vi "SOFandEOF_del.vi"(8 "error in (no error)":errorcluster, 11 "ISO 14443 B UP in":refnum<class "ISO 14443 B UP.lvclass">) -> (0 "error out":errorcluster, 3 "ISO 14443 B UP out":refnum<class "ISO 14443 B UP.lvclass">)   [LabVIEW 2019, in "ISO 14443 B UP.lvclass"]
uses:
  ISO 14443 B UP.lvclass
  TypeDef/Store.ctl
  ISO 14443 B UP.lvclass/ISO 14443 B UP.ctl
  RFID system.lvclass
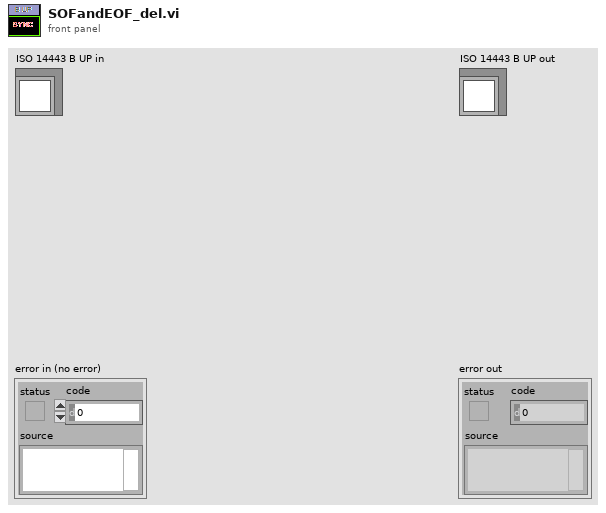
[diagram p1: front panel]
types:
  T1 = typedef "Store.ctl" = enum16{"envelope", "noise", "demSubCar", "CH_frame", "Decode", "demodulate", "in", "out", "sum", "subCarrier", "frame", "command", "encode", "modulate", "encode_UP", "modulate_up", "demod_up", "envelop_up", "sum_up", "out_up", "in_up"}
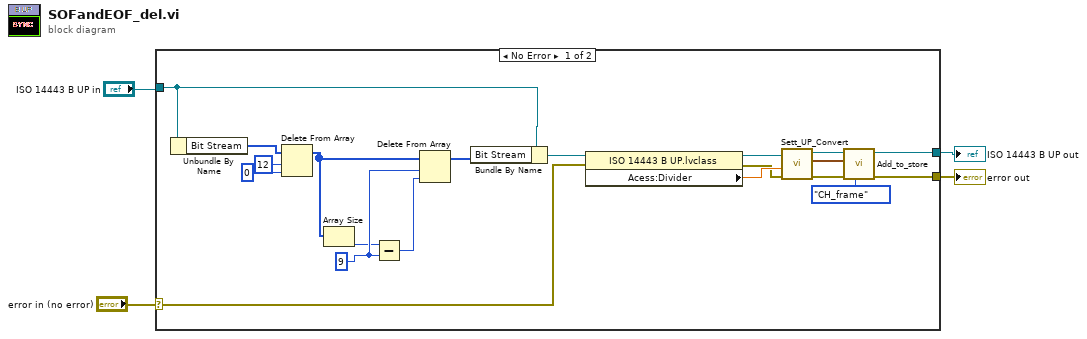
[diagram p0: block diagram]
diagram:
  n1 = case shown="No Error" "error in (no error)" {
    selector: "error in (no error)" -> [w6 w25]
    tunnel: "ISO 14443 B UP in" -> [w16 w26]
    tunnel: [w13 w26] -> w1
    tunnel: [w11 w25] -> w2
    frame No Error {
      w22 = 9 ("length")
      n2 = Unbundle By Name(w16) -> ("Bit Stream"=w18:u8[])
      n3 = Delete From Array(array=w18, length=12, index=0) -> (array with subset deleted=w24:u8[])  [unwired: 1 out]
      n4 = Array Size(array=w24) -> (size(s)=w20:i32)
      n5 = Subtract(x=w20, y=w22) -> (x-y=w21:i32)
      n6 = Delete From Array(array=w24, length=w22, index=w21) -> (array with subset deleted=w17:u8[])  [unwired: 1 out]
      n7 = Bundle By Name(cluster=w16, "Bit Stream"=w17) -> (w15:refnum<class "ISO 14443 B UP.lvclass">)
      n8 = property class="ISO 14443 B UP.lvclass"(reference=w15, error in=w6) -> (reference out=w8:refnum<class "ISO 14443 B UP.lvclass">, error out=w5:errorcluster, "Acess:Divider"=w7:dbl)
      n9 = call-dynamic "Sett_UP_Convert.vi"("error in (no error)"=w5, "Divider(1)"=w7, "ISO 14443 B UP in"=w8) -> ("error out"=w12:errorcluster, "Waveform"=w9:waveform(dbl), "ISO 14443 B UP out"=w14:refnum<class "ISO 14443 B UP.lvclass">)  [unwired: 6 in]
      n10 = call "Add_to_store.vi"("Store"=Store."CH_frame", "error in (no error)"=w12, "Waveform"=w9, "RFID system in"=w14) -> ("error out"=w11:errorcluster, "RFID system out"=w13:refnum<class "ISO 14443 B UP.lvclass">)  [unwired: 6 in]
    }
    frame Error {
    }
  }
  "error out" <- w2
  "ISO 14443 B UP out" <- w1
